vi "Calc HPF DWORD Size.vi"(4 "Profile Info":T1) -> (1 "DWORD Size":u32)   [LabVIEW 2014, in "Keyence LJ-V7000.lvlib"]
uses:
  Keyence LJ-V7000.lvlib
  Public/Clusters/Profile Info.ctl
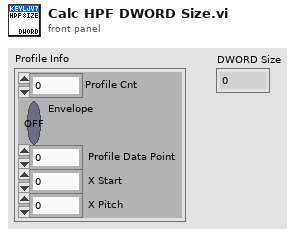
[diagram p1: front panel]
types:
  T1 = typedef "Keyence LJ-V7000.lvlib/Profile Info.ctl" = cluster{"Profile Cnt":u8, "Envelope":bool, " Profile Data Point":u16, " X Start":i32, " X Pitch":i32}
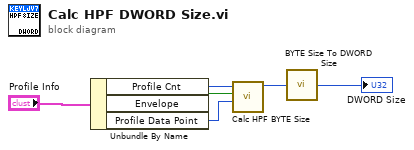
[diagram p0: block diagram]
diagram:
  n1 = Unbundle By Name("Profile Info") -> ("Profile Cnt"=w1:u8, "Envelope"=w2:bool, "Profile Data Point"=w3:u16)
  n2 = call "Calc HPF BYTE Size.vi"("Profile Data Point"=w3, "Envelope"=w2, "Profile Cnt"=w1) -> ("Profile Size"=w4:u32)  [unwired: 8 in]
  n3 = call "BYTE Size To DWORD Size.vi"("BYTE Size"=w4) -> ("DWORD Size"=→"DWORD Size":u32)
